vi "5.LM35 Sensor.vi"() -> ()   [LabVIEW 2014]
uses:
  <vilib>/LabVIEW Interface for Arduino/LabVIEW Interface for Arduino.lvlib
panel:
  out "Waveform Chart":dbl(graph)
  out "Slide":dbl(slide) scale=0.0..100.0
  in  "VISA resource":refnum<visa-resource-name>
  in  "Analog Input Pin (0)":u8
  in  "?":bool
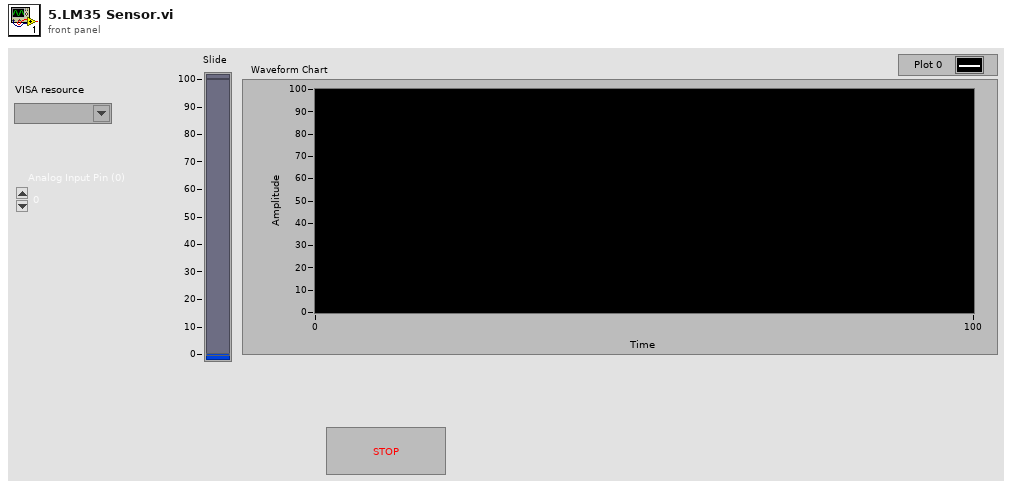
[diagram p1: front panel]
types:
  T1 = typedef "LabVIEW Interface for Arduino.lvlib/Arduino Resource.ctl" = cluster{"VISA resource":refnum<visa-resource-name>, "Board Type":T2, "Connection Type":enum8{"USB / Serial"}, "Bytes Per Packet (15)":u8}
  T2 = typedef "LabVIEW Interface for Arduino.lvlib/Board Type.ctl" = enum16{"Uno", "Dimuelanove w/Atmega 328", "Mega 2560"}
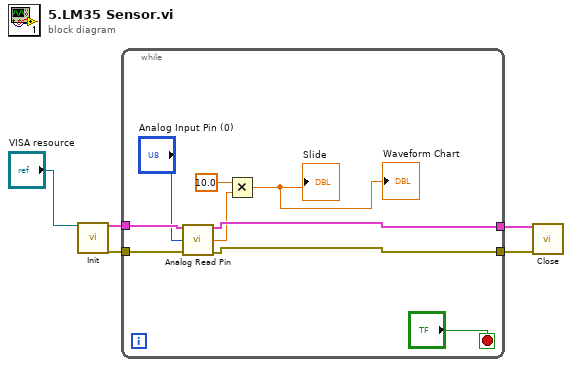
[diagram p0: block diagram]
diagram:
  n1 = call <vilib>:"Init.vi"("VISA resource"="VISA resource") -> ("Arduino Resource"=w5:T1, "error out"=w3:errorcluster)  [unwired: 17 in]
  n2 = while {
    tunnel: w5 -> [w13]
    tunnel: [w10] -> w4
    tunnel: w3 -> [w12]
    tunnel: [w9] -> w2
    stop <- "?" stop-if-true
    n3 = call <vilib>:"Analog Read Pin.vi"("Arduino Resource"=w13, "Analog Input Pin (0)"="Analog Input Pin (0)", "error in"=w12) -> ("Arduino Resource"=w10:T1, "Voltage"=w8:dbl, "error out"=w9:errorcluster)  [unwired: 10 in]
    n4 = Multiply(x=10.0, y=w8) -> (x*y=→"Slide" →"Waveform Chart":dbl)
  }
  n5 = call <vilib>:"Close.vi"("Arduino Resource"=w4, "error in"=w2) -> ()  [unwired: 13 in, 1 out]
